vi "ZGenerate.vi"() -> ()   [LabVIEW 2016]
uses:
  <vilib>/Analysis/NI_AALPro.lvlib
  <vilib>/Analysis/polynomials.llb/Unique Numbers and Multiplicity (DBL).vi
panel:
  in  "IV file name":string="decimated_21-BG+SG_Sweep+OVERNIGHT"
  in  "Processed data folder":path=path "B:/SketchSET/SA03008H.20180718/processed"
  in  "# of fields/Temperatures":i32=1
  in  "Field Period":i32=1
  in  "File or Folder Path":path=path "B:/SketchSET/SA03008H.20180718/21-BG+SG_Sweep+OVERNIGHT"
  in  "Additional comments":string
  in  "IV setup":T1={"# of Vslow"=101, "# Vfast"=41, "#IV Curves at each gate"=1, "B/T offset"=0, "Discard first # curves"=0, "Manual offset"=0}
  in  "Scan names":string[](array[string])=["DSA_Vsg1", "B", "B"]
  in  "Portion of data":cluster{dbl, dbl}(slide)={1.0, 0.0} scale=0.0..1.0
  in  "Decimate point":dbl=10.0 format="%#_1f"
  in  "T/B     third axis":bool
  in  "Extract parameters from comments?":bool=TRUE
  in  "index 2":T2={"A"=3, "B"=5, "C"=3, "D"=5, "E"=3, "N1"=2, "N2"=2, "N3"=3, "N4"=4, "A 1"=3, "A 2"=3, "C 1"=3, "C 2"=3, "E 2"=4}
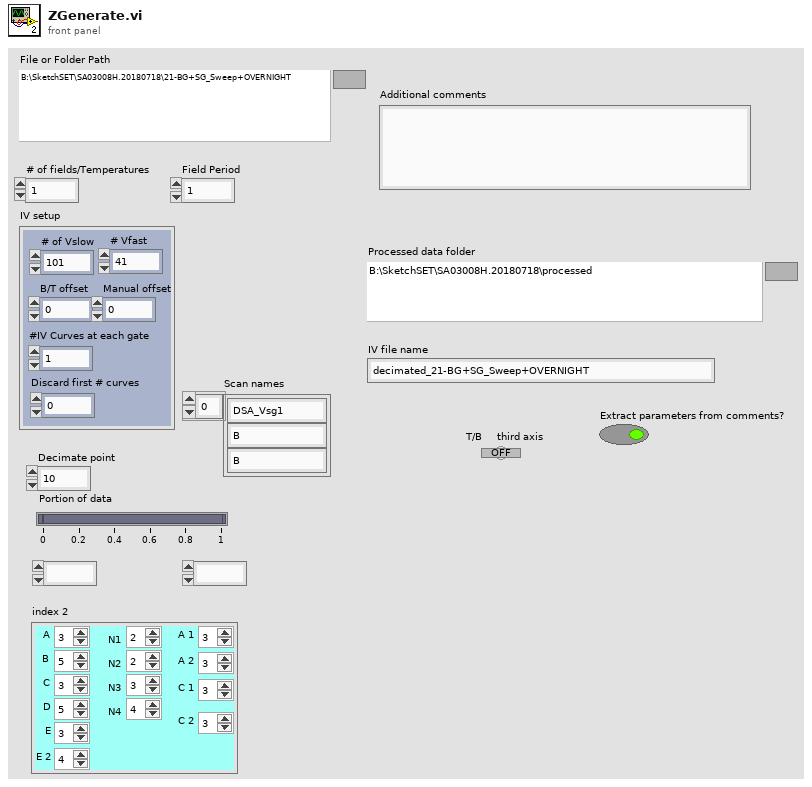
[diagram p1: front panel]
types:
  T1 = cluster{"# of Vslow":i32, "# Vfast":i32, "#IV Curves at each gate":i32, "B/T offset":i32, "Discard first # curves":i32, "Manual offset":i32}
  T2 = cluster{"A":i32, "B":i32, "C":i32, "D":i32, "E":i32, "N1":i32, "N2":i32, "N3":i32, "N4":i32, "A 1":i32, "A 2":i32, "C 1":i32, "C 2":i32, "E 2":i32}
  T3 = enum16{"open", "replace", "create", "open or create", "replace or create", "replace or create with confirmation"}
  T4 = typedef "SweepControl.lvclass/ScanControl.ctl" = T5[]
  T5 = typedef "SweepControl.lvclass/Cluster - ScanControl.ctl" = cluster{"Priority":T6, "Scan name":T7}
  T6 = typedef "SweepControl.lvclass/Enum - Priority.ctl" = enum16{"Priority 0", "Priority 1", "Priority 2", "Priority 3", "Priority 4", "Priority 5"}
  T7 = typedef "SweepControl.lvclass/Enum - Action.ctl" = enum16{"OFF", "DSA_Vamp", "DSA_freq", "DSA_Vsg1", "DSA_Vsg2", "DSA_Vsg3", "DAQ_Vbg", "B_Field", "Humidity", "Temp", "MW_freq1", "MW_freq2", "MW_amplitude1", "MW_amplitude2"}
  T8 = typedef "SweepControl.lvclass/ScanParamters.ctl" = T9[]
  T9 = typedef "SweepControl.lvclass/Cluster - ScanParamters.ctl" = cluster{"Start":dbl, "End":dbl, "Step":dbl, "Rate":dbl, "wait (ms)":u32, "address":refnum<visa-resource-name>, "Channel":i32}
  T10 = cluster{"Sorted scan control":cluster{T4}[], "Sorted scan parameters":cluster{T8}[], "# Of Sweep Pts. Fast to Slow":i16[]}
  T11 = cluster{"IV":cluster{dbl[], dbl[]}[][][], "IV-2T":cluster{dbl[], dbl[]}[][][], "Vfast":dbl[][], "Vslow":dbl[], dbl[], string, "Scan names":string[]}
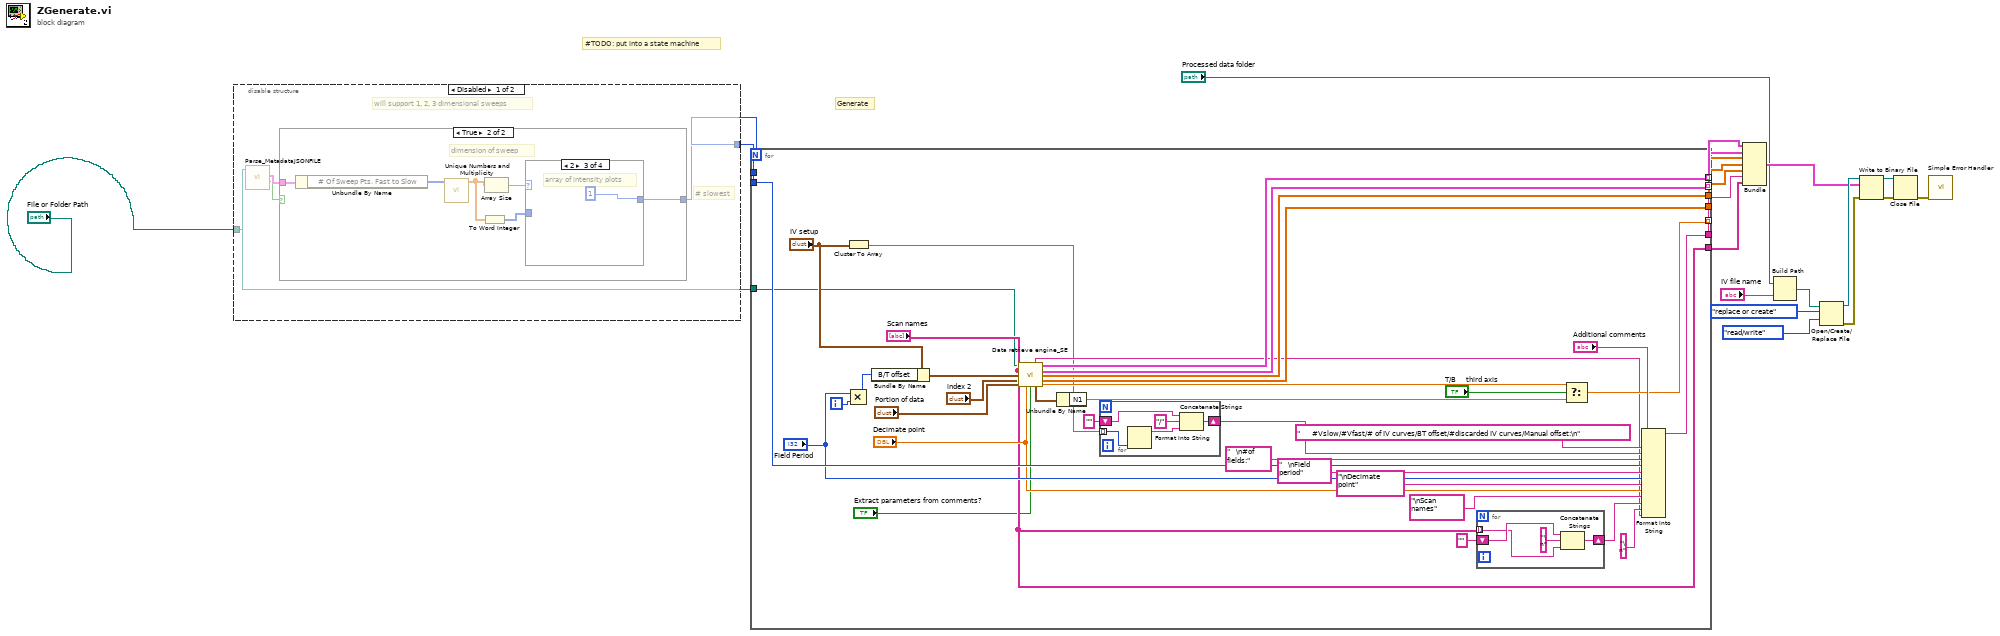
[diagram p0: block diagram]
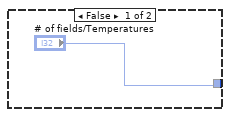
[diagram p2: hidden frame]
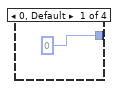
[diagram p3: hidden frame]
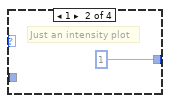
[diagram p4: hidden frame]
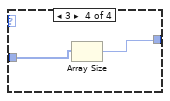
[diagram p5: hidden frame]
diagram:
  # "#TODO: put into a state machine"
  # "Generate"
  n1 = disable-structure shown="Disabled" {
    disable-tunnel: [w23 _] -> w2
    disable-tunnel: "File or Folder Path" -> [w21 _]
    frame Disabled {
      # "will support 1, 2, 3 dimensional sweeps"
      # "# slowest"
      n2 = call "Parse_MetadataJSONFILE.vi"("File or Folder Path"=w21) -> ("file or folder exists?"=w22:bool, "output cluster"=w24:T10)  [unwired: 8 in, 1 out]
      n3 = case shown="True" w22 {
        tunnel: w24 -> [_ w31]
        tunnel: ["# of fields/Temperatures" w28] -> w23
        frame False {
        }
        frame True {
          # "dimension of sweep"
          n4 = Unbundle By Name(w31) -> ("# Of Sweep Pts. Fast to Slow"=w30:i16[])
          n5 = call-poly <vilib>:"Unique Numbers and Multiplicity.vi"("Numbers"=w30) -> ("Unique Numbers"=w27:dbl[])  [unwired: 8 in, 2 out]
          n6 = To Word Integer(number=w27) -> (16bit integer=w26:i16[])
          n7 = Array Size(array=w27) -> (size(s)=w29:i32)
          n8 = case shown="2" w29 {
            tunnel: [0 1 1 w36] -> w28
            tunnel: w26 -> [_ _ _ w35]
            frame 0, Default {
            }
            frame 1 {
              # "Just an intensity plot"
            }
            frame 2 {
              # "array of intensity plots"
            }
            frame 3 {
              n9 = Array Size(array=w35) -> (size(s)=w36:i32)
            }
          }
        }
      }
    }
    frame Enabled {
    }
  }
  n10 = for {
    N: w2 -> [_]
    tunnel: [w71] -> w20 mode=indexing
    tunnel: [w67] -> w7
    tunnel: [w66] -> w6
    tunnel: [w65] -> w9 mode=indexing
    tunnel: [w48] -> w5 mode=indexing
    tunnel: w2 -> [_]
    tunnel: w2 -> [w56]
    tunnel: [w47] -> w8
    tunnel: ["Scan names"] -> w4
    tunnel: "File or Folder Path" -> [w38]
    i -> [w70]
    n11 = Multiply(x="Field Period", y=w70) -> (x*y=w68:i32)
    n12 = Cluster To Array(cluster="IV setup") -> (array=w37:i32[])
    n13 = Bundle By Name(cluster="IV setup", "B/T offset"=w68) -> (w61:T1)
    n14 = call "Data retrieve engine_SE.vi"("File or Folder Path"=w38, "Scan names"="Scan names", "IV setup"=w61, "index"="index 2", "Portion of data"="Portion of data", "Decimate point"="Decimate point", "Extract paramaters from comments?"="Extract parameters from comments?") -> ("Comments"=w42:string, "IV"=w71:cluster{dbl[], dbl[]}[][], "IV-2T"=w65:cluster{dbl[], dbl[]}[][], "Vfast"=w67:dbl[][], "Vslow"=w66:dbl[], "N"=w69:cluster{"N1":dbl, "N2":dbl, "N3":dbl, "N4":dbl}, "Vslowest"=w51:dbl)  [unwired: 2 in]
    n15 = Unbundle By Name(w69) -> ("N1"=w50:dbl)
    n16 = for {
      tunnel: w37 -> [w80] mode=indexing
      shift-right: [w77] -> w58
      shift-left: "" -> [w76]
      n17 = Format Into String(w80) -> (resulting string=w79:string)  [unwired: 3 in, 1 out]
      n18 = Concatenate Strings(w76, "/" ("string"), w79) -> (w77:string)
    }
    n19 = for {
      tunnel: "Scan names" -> [w73] mode=indexing
      shift-right: [w75] -> w44
      shift-left: "" -> [w74]
      n20 = Concatenate Strings(w74, "\n" ("string"), w73) -> (w75:string)
    }
    n21 = Select(t=w51, s="T/B     third axis", f=w50) -> (s? t:f=w48:dbl)
    n22 = Format Into String(initial string="Additional comments", "      #Vslow/#Vfast/# of IV curves/BT offset/#discarded IV curves/Manual offset:\n" ("string"), w58, "   \n#of fields:" ("string"), w56, "   \nField period" ("string"), "Field Period", "\nDecimate point", "Decimate point", "\nScan names", w44, "\n" ("input 11"), w42) -> (resulting string=w47:string)  [unwired: 2 in, 1 out]
  }
  n23 = Bundle("IV"=w20, "IV-2T"=w9, "Vfast"=w7, "Vslow"=w6, w5, w8, "Scan names"=w4) -> (w10:T11)  [unwired: 1 in]
  n24 = Build Path(base path="Processed data folder", name or relative path="IV file name") -> (appended path=w11:path)
  n25 = Open/Create/Replace File(file path (use dialog)=w11, operation (0:open)=T3."replace or create", access (0:read/write)=enum16{"read/write", "read-only", "write-only"}."read/write") -> (refnum out=w15:refnum<file>, error out=w16:errorcluster)  [unwired: 3 in, 1 out]
  n26 = Write to Binary File(file (use dialog)=w15, data=w10, error in=w16) -> (refnum out=w19:refnum<file>, error out=w18:errorcluster)  [unwired: 3 in, 1 out]
  n27 = Close File(refnum=w19, error in=w18) -> (error out=w17:errorcluster)  [unwired: 1 out]
  n28 = call <vilib>:"Simple Error Handler.vi"("error in (no error)"=w17) -> ()  [unwired: 4 in, 5 out]
